vi "Simulator.vi"() -> ()   [LabVIEW 2011]
panel:
  in  "Tab Control":T1(tab)
  in  "Initial Boat Location (x)":dbl=10.0
  in  "Initial Boat Location (y)":dbl=10.0
  in  "Waypoint Location (x)":dbl=16.0
  in  "Waypoint Location (y)":dbl=16.0
  in  "Absolute Wind Dir":i32(knob)=45 scale=-180.0..180.0
  in  "Initial Boat Heading":i32(knob) scale=-180.0..180.0
  in  "Loop delay (ms)":u32=100
  in  "v*dt":dbl=0.1
  out "Loop Iteration":i32
  out "Boat Path":cluster{"X":dbl, "Y":dbl}[](graph)
  out "Boat Location (y)":dbl
  out "Boat Location (x)":dbl
  out "Absolute heading\ntowards wpt":dbl
  out "dx and dy":cluster{"X":dbl, "Y":dbl}
  out "Distance to waypt":cluster{"X":dbl, "Y":dbl}
  out "New heading":i32(knob) scale=-180.0..180.0
  out "Apparent Wind Dir":i32(knob) scale=-180.0..180.0
  out "Last Heading":i32
  in  "stop":bool
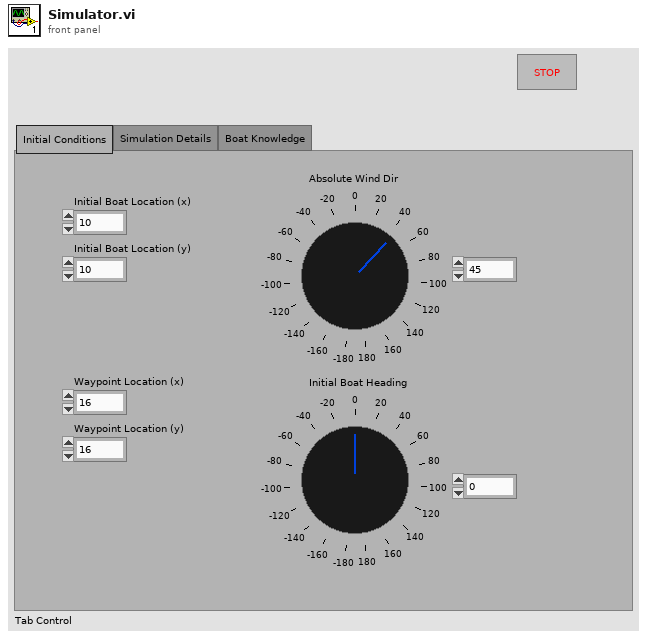
[diagram p1: front panel]
types:
  T1 = enum32{"Initial Conditions", "Simulation Details", "Boat Knowledge"}
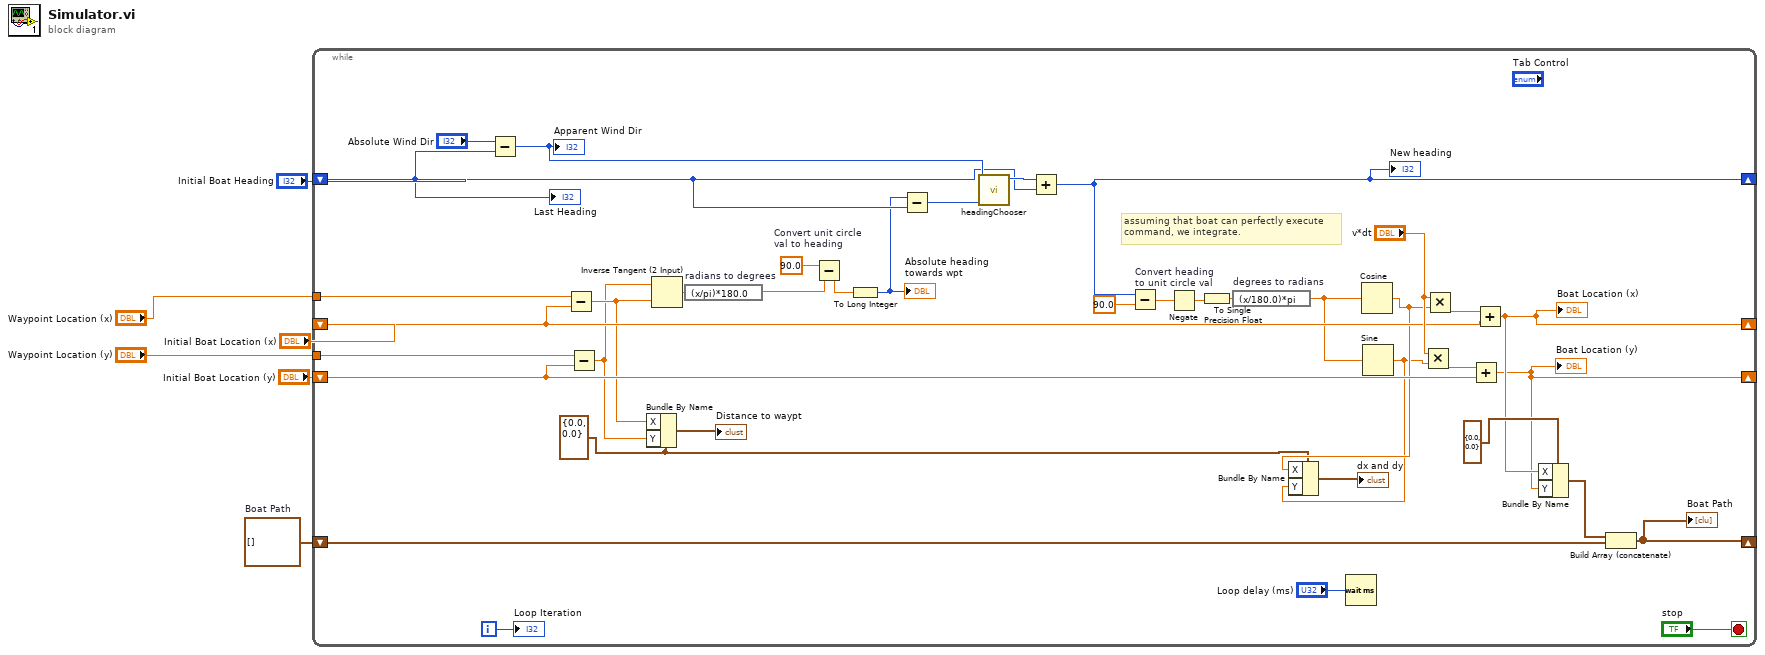
[diagram p0: block diagram]
diagram:
  w1 = cluster{"X":dbl, "Y":dbl}[] []  # Boat Path
  n1 = while {
    shift-right: [w35] -> _
    shift-left: "Initial Boat Location (x)" -> [w39]
    shift-right: [w34] -> _
    shift-left: "Initial Boat Location (y)" -> [w38]
    tunnel: "Waypoint Location (x)" -> [w41]
    tunnel: "Waypoint Location (y)" -> [w40]
    shift-right: [w10] -> _
    shift-left: "Initial Boat Heading" -> [w19]
    shift-right: [w32] -> _
    shift-left: w1 -> [w31]
    i -> [w29]
    stop <- "stop" stop-if-true
    w21 = cluster{"X":dbl, "Y":dbl} {"X"=0.0, "Y"=0.0} ("Cluster")
    # "assuming that boat can perfectly execute\ncommand, we integrate."
    n2 = Subtract(x="Absolute Wind Dir", y=w19) -> (x-y=w45:i32)
    "Apparent Wind Dir" <- w45
    n3 = Subtract(x=w41, y=w39) -> (x-y=w16:dbl)
    n4 = Subtract(x=w40, y=w38) -> (x-y=w15:dbl)
    n5 = Bundle By Name(cluster=w21, "X"=w16, "Y"=w15) -> (→"Distance to waypt":cluster{"X":dbl, "Y":dbl})
    n6 = Inverse Tangent (2 Input)(1:w16, 2:w15) -> (0:w17:dbl)
    n7 = expression code="(x/pi)*180.0" "radians to degrees"(w17) -> (w13:dbl)
    n8 = Subtract "Convert unit circle\nval to heading"(x=90.0, y=w13) -> (x-y=w14:dbl)
    n9 = To Long Integer(number=w14) -> (32bit integer=w18:i32)
    "Absolute heading\ntowards wpt" <- w18
    n10 = Subtract(x=w18, y=w19) -> (x-y=w37:i32)
    n11 = call "headingChooser.vi"("Waypoint Direction (relative to current heading)"=w37, "Wind Direction (relative to current heading)"=w45) -> ("Best Angle"=w20:i32)  [unwired: 9 in]
    n12 = Add(x=w20, y=w19) -> (x+y=w10:i32)
    "New heading" <- w10
    n13 = Subtract "Convert heading \nto unit circle val"(x=w10, y=90.0 ("x")) -> (x-y=w8:dbl)
    n14 = Negate(x=w8) -> (-x=w9:dbl)
    n15 = To Single Precision Float(number=w9) -> (single precision float=w25:sgl)
    n16 = expression code="(x/180.0)*pi" "degrees to radians"(w25) -> (w26:sgl)
    n17 = Wait (ms)(milliseconds to wait="Loop delay (ms)") -> ()  [unwired: 1 out]
    n18 = Cosine(x=w26) -> (cos(x)=w23:sgl)
    n19 = Sine(x=w26) -> (sin(x)=w22:sgl)
    n20 = Bundle By Name(cluster=w21, "X"=w23, "Y"=w22) -> (→"dx and dy":cluster{"X":dbl, "Y":dbl})
    n21 = Multiply(x="v*dt", y=w22) -> (x*y=w44:dbl)
    n22 = Multiply(x="v*dt", y=w23) -> (x*y=w43:dbl)
    n23 = Add(x=w44, y=w38) -> (x+y=w34:dbl)
    "Boat Location (y)" <- w34
    n24 = Add(x=w43, y=w39) -> (x+y=w35:dbl)
    "Boat Location (x)" <- w35
    n25 = Bundle By Name(cluster=cluster{"X":dbl, "Y":dbl} {"X"=0.0, "Y"=0.0}, "X"=w35, "Y"=w34) -> (w33:cluster{"X":dbl, "Y":dbl})
    n26 = Build Array (concatenate)(w33, w31) -> (w32:cluster{"X":dbl, "Y":dbl}[])
    "Boat Path" <- w32
    "Loop Iteration" <- w29
    "Last Heading" <- w19
  }
